vi "main_BRBcase.vi"() -> ()   [LabVIEW 2016]
uses:
  INPUTS.ctl
  <vilib>/DAQmx/read.llb/DAQmx Read (Analog 2D DBL NChan NSamp).vi
  <vilib>/DAQmx/configure/timing.llb/DAQmx Timing (Sample Clock).vi
  <vilib>/DAQmx/miscellaneous.llb/DAQmx Fill In Error Info.vi
panel:
  out "I_CELL":dbl format="%0.2f"
  out "I_LOAD":dbl format="%0.2f"
  out "I_PV":dbl format="%0.2f"
  out "V_CELL":dbl format="%0.2f"
  out "V_BUS":dbl format="%0.2f"
  out "Currents":cluster{dbl[], dbl[]}[](graph) caption="VCC"
  out "Voltages":cluster{dbl[], dbl[]}[](graph) caption="VCC"
  in  "stop":bool
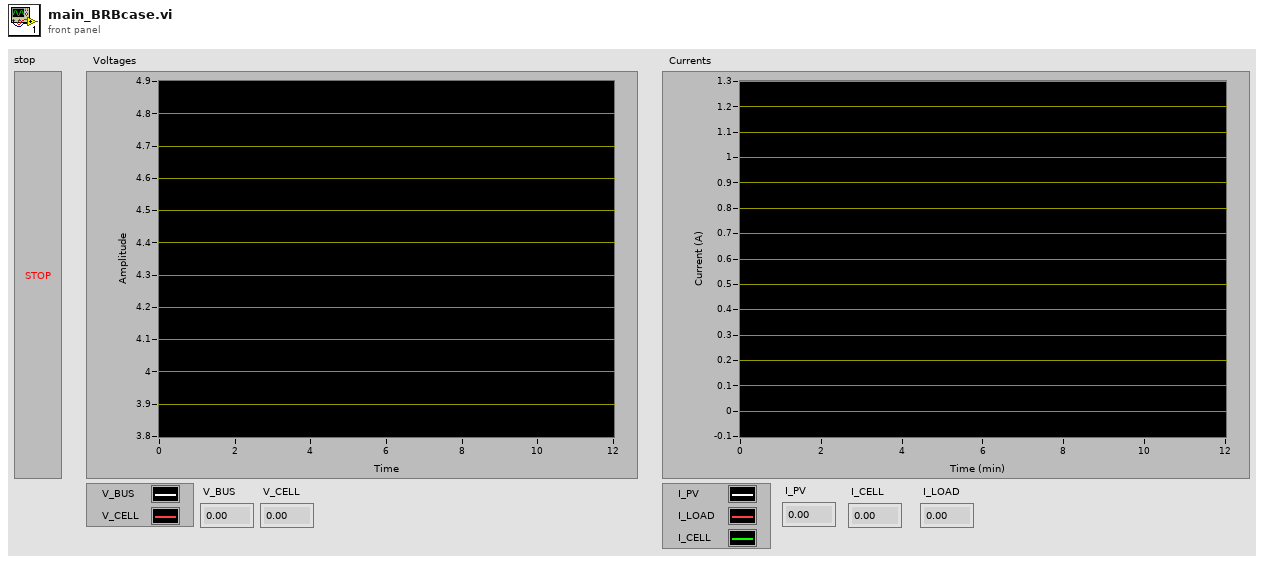
[diagram p1: front panel]
types:
  T1 = enum16{"open", "open or create", "create or replace", "create", "open (read only)"}
  T2 = typedef "INPUTS.ctl" = enum16{"VCC", "I_PV", "I_LOAD", "I_CELL", "V_BUS", "V_CELL"}
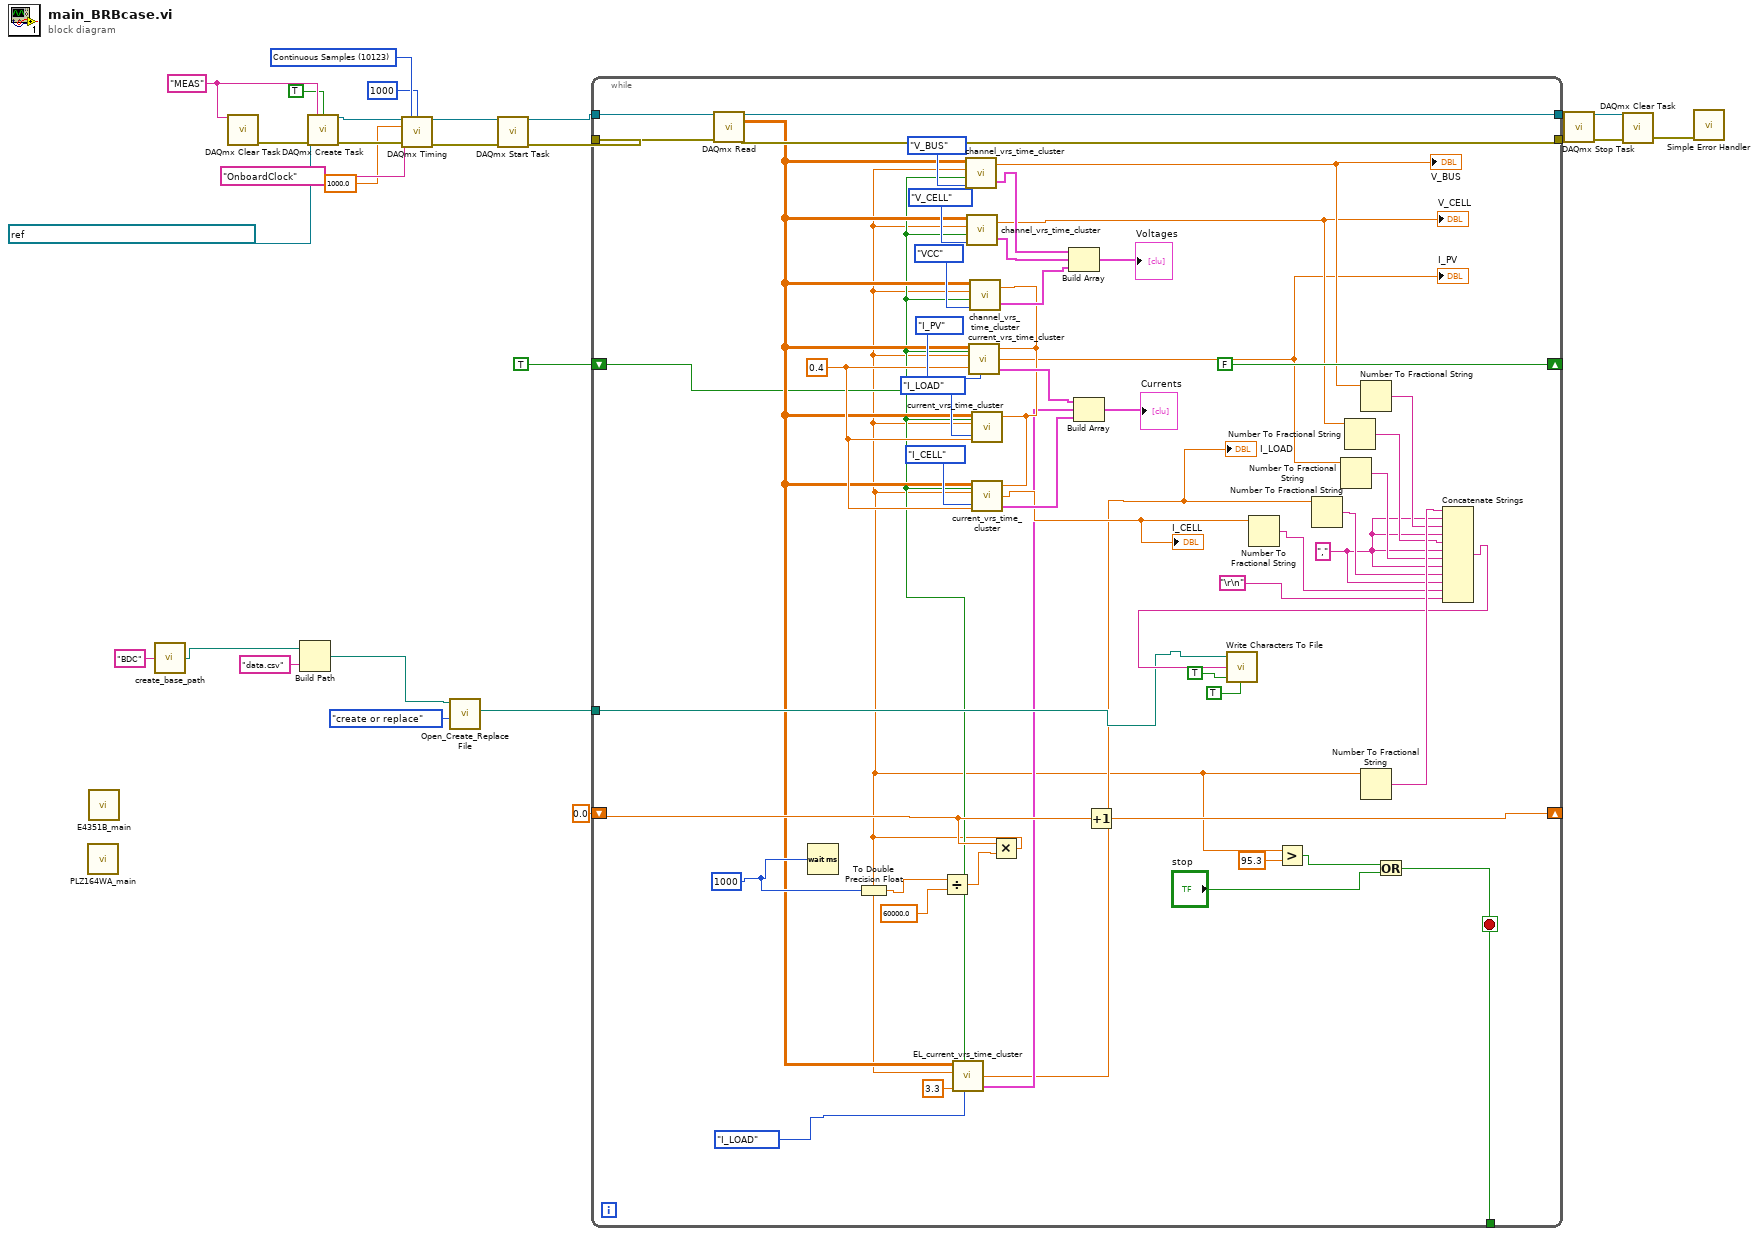
[diagram p0: block diagram]
diagram:
  w22 = 10123 items=["Finite Samples"=10178, "Continuous Samples"=10123, "Hardware Timed Single Point"=12522] ("sample mode")
  w9 = "MEAS" ("new task name")
  n1 = call "PLZ164WA_main.vi"() -> ()  [unwired: 12 in]
  n2 = call "E4351B_main.vi"() -> ()  [unwired: 1 in]
  n3 = call "create_base_path.vi"("project name"="BDC") -> ("base path"=w3:path)
  n4 = call <vilib>:"DAQmx Clear Task.vi"("task in"=w9) -> ("error out"=w10:errorcluster)  [unwired: 14 in]
  n5 = Build Path(base path=w3, name or relative path="data.csv") -> (appended path=w5:path)
  n6 = call <vilib>:"DAQmx Create Task.vi"("new task name"=w9, "auto cleanup"=TRUE, "global virtual channels"=refnum<k21> "VCC, I_PV, I_LOAD, I_CELL, V_BUS, V_CELL", "error in"=w10) -> ("task out"=w24:refnum<k21>, "error out"=w23:errorcluster)  [unwired: 10 in]
  n7 = call-poly <vilib>:"DAQmx Timing.vi"("task/channels in"=w24, "sample mode"=w22, "samples per channel"=1000, "rate"=1000.0, "source"=tag "OnboardClock", "error in"=w23) -> ("task out"=w19:refnum<k21>, "error out"=w18:errorcluster)  [unwired: 8 in]
  n8 = call <vilib>:"Open_Create_Replace File.vi"("function (open:0)"=T1."create or replace", "file path"=w5) -> ("new file path"=w1:path)  [unwired: 6 in, 3 out]
  n9 = call <vilib>:"DAQmx Start Task.vi"("task/channels in"=w19, "error in"=w18) -> ("task out"=w17:refnum<k21>, "error out"=w16:errorcluster)  [unwired: 12 in]
  n10 = while {
    shift-right: [w39] -> _
    shift-left: 0.0 -> [w40]
    shift-right: [FALSE ("Clear Graph?")] -> _
    shift-left: TRUE ("Clear Graph?") -> [w37]
    tunnel: w17 -> [w75]
    tunnel: w16 -> [w74]
    tunnel: [w73] -> w15
    tunnel: [w72] -> w14
    tunnel: w1 -> [w41]
    tunnel: [w28] -> _
    stop <- w28 stop-if-true
    w44 = "," ("string")
    w58 = 0.4 ("sensitivity (V/A)")
    w76 = u32 1000 ("milliseconds to wait")
    n11 = call-poly <vilib>:"DAQmx Read.vi"("task/channels in"=w75, "error in"=w74) -> ("task out"=w73:refnum<k21>, "data"=w38:dbl[][], "error out"=w72:errorcluster)  [unwired: 11 in]
    n12 = Wait (ms)(milliseconds to wait=w76) -> ()  [unwired: 1 out]
    n13 = To Double Precision Float(number=w76) -> (double precision float=w79:dbl)
    n14 = Divide(x=w79, y=60000.0) -> (x/y=w77:dbl)
    n15 = Multiply(x=w40, y=w77) -> (x*y=w32:dbl)
    n16 = call "EL_current_vrs_time_cluster.vi"("Input data"=w38, "Clear Graph?"=w37, "Time"=w32, "Enum"=INPUTS."I_LOAD", "sensitivity (V/A)"=3.3) -> ("rms value"=w33:dbl, "Cluster"=w34:cluster{dbl[], dbl[]})  [unwired: 2 in]
    "I_LOAD" <- w33
    n17 = call "channel_vrs_time_cluster.vi"("Enum"=INPUTS."V_BUS", "Clear Graph?"=w37, "Time"=w32, "Input data"=w38) -> ("Cluster"=w69:cluster{dbl[], dbl[]}, "rms value"=w53:dbl)
    "V_BUS" <- w53
    n18 = call "channel_vrs_time_cluster.vi"("Enum"=INPUTS."V_CELL", "Clear Graph?"=w37, "Time"=w32, "Input data"=w38) -> ("Cluster"=w68:cluster{dbl[], dbl[]}, "rms value"=w52:dbl)
    "V_CELL" <- w52
    n19 = call "channel_vrs_time_cluster.vi"("Enum"=INPUTS."VCC", "Clear Graph?"=w37, "Time"=w32, "Input data"=w38) -> ("Cluster"=w66:cluster{dbl[], dbl[]}, "rms value"=w57:dbl)
    n20 = call "current_vrs_time_cluster.vi"("Input data"=w38, "Clear Graph?"=w37, "Time"=w32, "Enum"=INPUTS."I_PV", "sensitivity (V/A)"=w58, "VCC"=w57) -> ("rms value"=w51:dbl, "Cluster"=w60:cluster{dbl[], dbl[]})  [unwired: 1 in]
    "I_PV" <- w51
    n21 = call "current_vrs_time_cluster.vi"("Input data"=w38, "Clear Graph?"=w37, "Time"=w32, "Enum"=INPUTS."I_LOAD", "sensitivity (V/A)"=w58, "VCC"=w57) -> ()  [unwired: 1 in, 2 out]
    n22 = call "current_vrs_time_cluster.vi"("Input data"=w38, "Clear Graph?"=w37, "Time"=w32, "Enum"=INPUTS."I_CELL", "sensitivity (V/A)"=w58, "VCC"=w57) -> ("rms value"=w50:dbl, "Cluster"=w59:cluster{dbl[], dbl[]})  [unwired: 1 in]
    "I_CELL" <- w50
    n23 = Build Array(w69, w68, w66) -> (→"Voltages":cluster{dbl[], dbl[]}[])
    n24 = Build Array(w60, w34, w59) -> (→"Currents":cluster{dbl[], dbl[]}[])
    n25 = Increment(x=w40) -> (x+1=w39:dbl)
    n26 = Number To Fractional String(number=w50) -> (F-format string=w43:string)  [unwired: 3 in]
    n27 = Greater?(x=w32, y=95.3) -> (0:w29:bool)
    n28 = Number To Fractional String(number=w33) -> (F-format string=w45:string)  [unwired: 3 in]
    n29 = Number To Fractional String(number=w51) -> (F-format string=w46:string)  [unwired: 3 in]
    n30 = Number To Fractional String(number=w52) -> (F-format string=w47:string)  [unwired: 3 in]
    n31 = Number To Fractional String(number=w53) -> (F-format string=w48:string)  [unwired: 3 in]
    n32 = Number To Fractional String(number=w32) -> (F-format string=w54:string)  [unwired: 3 in]
    n33 = Or(x=w29, y="stop") -> (x .or. y?=w28:bool)
    n34 = Concatenate Strings(w54, w44, w48, w44, w47, w44, w46, w44, w45, w44, w43, "\r\n") -> (w49:string)
    n35 = call <vilib>:"Write Characters To File.vi"("convert eol? (no:F)"=TRUE, "append to file? (new file:F)"=TRUE, "character string"=w49, "file path (dialog if empty)"=w41) -> ()  [unwired: 1 in, 1 out]
  }
  n36 = call <vilib>:"DAQmx Stop Task.vi"("task/channels in"=w15, "error in"=w14) -> ("task out"=w13:refnum<k21>, "error out"=w12:errorcluster)  [unwired: 12 in]
  n37 = call <vilib>:"DAQmx Clear Task.vi"("task in"=w13, "error in"=w12) -> ("error out"=w11:errorcluster)  [unwired: 13 in]
  n38 = call <vilib>:"Simple Error Handler.vi"("error in (no error)"=w11) -> ()  [unwired: 4 in, 5 out]
